vi "RSZVB Get Calibration Connector.vi"(8 "error in (no error)":errorcluster {"code" format="%.0x"}, 9 "Connector Name":string, 10 "Channel (1)":i32=1, 11 "VISA session":refnum<visa-resource-name>) -> (0 "error out":errorcluster {"code" format="%.0x"}, 1 "Propagation Mode":i32, 3 "dup VISA session":refnum<visa-resource-name>, 4 "Impedance":dbl format="%^.3e", 5 "Relative Permittivity":dbl format="%^.3e", 7 "Connector Type":i32)   [LabVIEW 2011]
doc: "This VI queries the user-defined connector types.\n\nRemote-control command(s):\n[SENSe<Ch>:]CORRection:CONNection? '<conn_name>'"
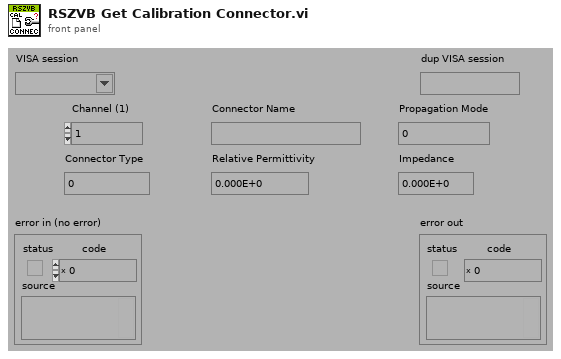
[diagram p1: front panel]
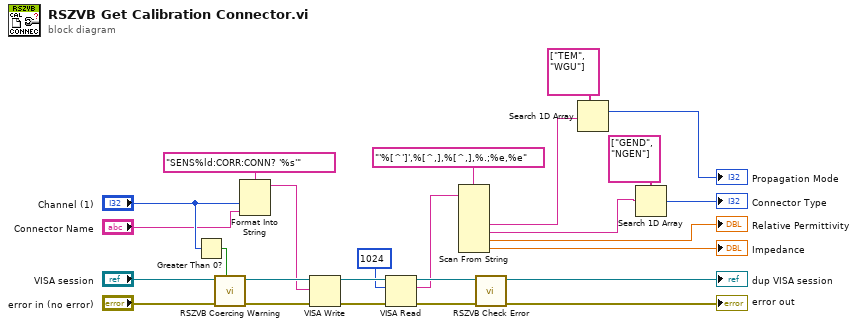
[diagram p0: block diagram]
diagram:
  n1 = Greater Than 0?(x="Channel (1)") -> (x > 0?=w20:bool)
  n2 = call "RSZVB Coercing Warning.vi"("In Range?"=w20, "error in (no error)"="error in (no error)", "VISA session"="VISA session") -> ("error out"=w25:errorcluster, "dup VISA session"=w26:refnum<visa-resource-name>)  [unwired: 7 in]
  n3 = Format Into String(format string="SENS%ld:CORR:CONN? '%s'", "Channel (1)", "Connector Name") -> (resulting string=w18:string)  [unwired: 2 in, 1 out]
  n4 = VISA Write(VISA resource name=w26, write buffer=w18, error in (no error)=w25) -> (VISA resource name out=w24:refnum<visa-resource-name>, error out=w23:errorcluster)  [unwired: 1 out]
  n5 = VISA Read(VISA resource name=w24, byte count=u32 1024 ("byte count (0)"), error in (no error)=w23) -> (VISA resource name out=w22:refnum<visa-resource-name>, read buffer=w1:string, error out=w21:errorcluster)  [unwired: 1 out]
  n6 = Scan From String(format string="'%[^']',%[^,],%[^,],%.;%e,%e", input string=w1) -> (output 2=w5:string, output 3=w4:string, output 4=→"Relative Permittivity":dbl, output 5=→"Impedance":dbl)  [unwired: 8 in, 3 out]
  n7 = call "RSZVB Check Error.vi"("error in (no error)"=w21, "VISA session"=w22) -> ("error out"=→"error out":errorcluster, "dup VISA session"=→"dup VISA session":refnum<visa-resource-name>)  [unwired: 8 in]
  n8 = Search 1D Array(1D array=string[] ["TEM", "WGU"] ("array 2"), element=w5) -> (index of element=→"Propagation Mode":i32)  [unwired: 1 in]
  n9 = Search 1D Array(1D array=string[] ["GEND", "NGEN"] ("array 2"), element=w4) -> (index of element=→"Connector Type":i32)  [unwired: 1 in]
